vi "saveTetTaskToMAX..vi"() -> ()   [LabVIEW 2010]
doc: "Author: Mani Subramaniyan\n2011-09-14\n\nThis vi assumes you have 7, 4498 cards for recording from tetrodes."
uses:
  <vilib>/DAQmx/create/channels.llb/DAQmx Create Channel (AI-Voltage-Basic).vi
  <vilib>/DAQmx/configure/timing.llb/DAQmx Timing (Sample Clock).vi
  <vilib>/imath/engines/lvmath2/RunTimeEngine/ErrorHandling/NIMS_Finalize Error.vi
  <vilib>/imath/engines/lvmath2/RunTimeEngine/RangeToken/NIMS_Range_R2 - Integer.vi
  <instcachedir>/0/NIMS_Range_R2 - Integer_217CA55F27D14E80B3D190635C7B3F47.lvgen/NIMS_Range_R2 - Integer_217CA55F27D14E80B3D190635C7B3F47_000.vi
  <vilib>/imath/engines/lvmath2/RunTimeEngine/NodeEndStatement/NIMS_NodeEndStatement_Output.vi
  <instcachedir>/0/NIMS_NodeEndStatement_Output_53EC0D466D134D7ABD903AC30B43404B.lvgen/NIMS_NodeEndStatement_Output_53EC0D466D134D7ABD903AC30B43404B_004.vi
  <vilib>/imath/engines/lvmath2/RunTimeEngine/CommandStatement/MC_CommandStatement_break.vi
  <vilib>/imath/engines/lvmath2/RunTimeEngine/VariableToken/NIMS_VariableToken_CondDefinedDefinedByReplace.vi
  <instcachedir>/0/NIMS_VariableToken_CondDefinedDefinedByReplace_D162CFFC24174562A9FEA619A91E1A56.lvgen/NIMS_VariableToken_CondDefinedDefinedByReplace_D162CFFC24174562A9FEA619A91E1A56_003.vi
  <vilib>/imath/engines/lvmath2/RunTimeEngine/ReplaceToken/NIMS_Replace - Check Linear.vi
  <instcachedir>/0/NIMS_Replace - Check Linear_662D5651E4E34E0584DA82A256193A4C.lvgen/NIMS_Replace - Check Linear_662D5651E4E34E0584DA82A256193A4C_006.vi
  <vilib>/imath/engines/lvmath2/RunTimeEngine/ReplaceToken/NIMS_Replace - Size Check _(_)=S.vi
  <instcachedir>/0/NIMS_Replace - Size Check _(_)=S_6CAC13ACC74349C582FDAB09BCDAB70F.lvgen/NIMS_Replace - Size Check _(_)=S_6CAC13ACC74349C582FDAB09BCDAB70F_005.vi
  <vilib>/imath/engines/lvmath2/RunTimeEngine/ReplaceToken/NIMS_Replace - V(S)=S.vi
  <instcachedir>/0/NIMS_Replace - V(S)=S_78FDB6CCD265407D8926E4CF958018EB.lvgen/NIMS_Replace - V(S)=S_78FDB6CCD265407D8926E4CF958018EB_003.vi
  <vilib>/imathl/engines/lvmath/Functions/Error Handling/Create Error.vi
  <instcachedir>/0/NIMS_VariableToken_CondDefinedDefinedByReplace_D162CFFC24174562A9FEA619A91E1A56.lvgen/NIMS_VariableToken_CondDefinedDefinedByReplace_D162CFFC24174562A9FEA619A91E1A56_002.vi
  <instcachedir>/0/NIMS_Replace - Check Linear_662D5651E4E34E0584DA82A256193A4C.lvgen/NIMS_Replace - Check Linear_662D5651E4E34E0584DA82A256193A4C_005.vi
  <vilib>/imath/engines/lvmath2/RunTimeEngine/VariableToken/Read/NIMS_Get Elements - SorM(_,_) - Check - Check.vi
  <instcachedir>/0/NIMS_Get Elements - SorM(_,_) - Check - Check_507509EC3FB3473FB85D8EE7246D3CED.lvgen/NIMS_Get Elements - SorM(_,_) - Check - Check_507509EC3FB3473FB85D8EE7246D3CED_005.vi
  <instcachedir>/0/NIMS_Replace - Size Check _(_)=S_6CAC13ACC74349C582FDAB09BCDAB70F.lvgen/NIMS_Replace - Size Check _(_)=S_6CAC13ACC74349C582FDAB09BCDAB70F_004.vi
  <instcachedir>/0/NIMS_Replace - V(S)=S_78FDB6CCD265407D8926E4CF958018EB.lvgen/NIMS_Replace - V(S)=S_78FDB6CCD265407D8926E4CF958018EB_002.vi
  <vilib>/imath/engines/lvmath2/RunTimeEngine/ErrorHandling/NIMS_Create Error From Enums.vi
  <vilib>/imath/engines/lvmath2/RunTimeEngine/VariableToken/NIMS_VariableToken_CondDefined.vi
  <instcachedir>/0/NIMS_VariableToken_CondDefined_40F5A17402C24691AFAF09F6009BF744.lvgen/NIMS_VariableToken_CondDefined_40F5A17402C24691AFAF09F6009BF744_004.vi
  <instcachedir>/0/NIMS_VariableToken_CondDefined_40F5A17402C24691AFAF09F6009BF744.lvgen/NIMS_VariableToken_CondDefined_40F5A17402C24691AFAF09F6009BF744_003.vi
  <vilib>/imath/engines/lvmath2/RunTimeEngine/BuiltInFunctions/transpose/NIMS_transpose(GM).vi
  <instcachedir>/0/NIMS_transpose(GM)_822C4B39CC3F4B34B360A85316D387F1.lvgen/NIMS_transpose(GM)_822C4B39CC3F4B34B360A85316D387F1_003.vi
  <vilib>/imath/engines/lvmath2/RunTimeEngine/VariableToken/Read/NIMS_Get Elements - M($).vi
  <instcachedir>/0/NIMS_Get Elements - M($)_A8F2A19C5154485F939AC006E49BBA6A.lvgen/NIMS_Get Elements - M($)_A8F2A19C5154485F939AC006E49BBA6A_004.vi
  <vilib>/imath/engines/lvmath2/RunTimeEngine/VariableToken/Read/NIMS_Get Elements - CV(_) - Check(_).vi
  <instcachedir>/0/NIMS_Get Elements - CV(_) - Check(_)_64AEF14B7A4641C2943F7B5E6C404257.lvgen/NIMS_Get Elements - CV(_) - Check(_)_64AEF14B7A4641C2943F7B5E6C404257_001.vi
  <instcachedir>/0/NIMS_Get Elements - CV(_) - Check(_)_64AEF14B7A4641C2943F7B5E6C404257.lvgen/NIMS_Get Elements - CV(_) - Check(_)_64AEF14B7A4641C2943F7B5E6C404257_000.vi
  <vilib>/imath/engines/lvmath2/RunTimeEngine/BuiltInFunctions/sort/NIMS_[2o]_sort(RColV,I32,Str).vi
  <instcachedir>/0/NIMS_[2o]_sort(RColV,I32,Str)_8C46B823F3A24849A9EF3A3AB0F8B237.lvgen/NIMS_[2o]_sort(RColV,I32,Str)_8C46B823F3A24849A9EF3A3AB0F8B237_001.vi
  <vilib>/imath/engines/lvmath2/RunTimeEngine/VariableToken/Read/NIMS_Get Elements - CV(_) - Check.vi
  <instcachedir>/0/NIMS_Get Elements - CV(_) - Check_8515505E2F3A4209803E127475018AE3.lvgen/NIMS_Get Elements - CV(_) - Check_8515505E2F3A4209803E127475018AE3_001.vi
  <vilib>/imath/engines/lvmath2/RunTimeEngine/BuiltInFunctions/ones/NIMS_V=ones(I32,I32).vi
  <vilib>/imath/engines/lvmath2/RunTimeEngine/RangeToken/NIMS_Range.vi
  <instcachedir>/0/NIMS_Range_1C63927E4E474DADACDA97C3F2261A11.lvgen/NIMS_Range_1C63927E4E474DADACDA97C3F2261A11_000.vi
  <vilib>/imath/engines/lvmath2/RunTimeEngine/BuiltInFunctions/repeatmx/NIMS_repeatmx(GM, I32, I32).vi
  <instcachedir>/0/NIMS_repeatmx(GM, I32, I32)_69DEE8FEFC4F4D9AB51BA55E85245ECE.lvgen/NIMS_repeatmx(GM, I32, I32)_69DEE8FEFC4F4D9AB51BA55E85245ECE_004.vi
  <instcachedir>/0/NIMS_Get Elements - M($)_A8F2A19C5154485F939AC006E49BBA6A.lvgen/NIMS_Get Elements - M($)_A8F2A19C5154485F939AC006E49BBA6A_005.vi
  <instcachedir>/0/NIMS_Get Elements - CV(_) - Check_8515505E2F3A4209803E127475018AE3.lvgen/NIMS_Get Elements - CV(_) - Check_8515505E2F3A4209803E127475018AE3_003.vi
panel:
  in  "Stop Without Saving":bool
  in  "Deselect All":bool
  in  "Save Task Now":bool
  in  "Select All":bool
  out "error out":errorcluster
  in  "Sampling Rate (Hz)":dbl=32000.0 format="%0.2f"
  out "Channel Names":string[](array[string])=["t10c4", "t1c4", "t10c3", "t1c3", "t10c2", "t1c2", "t10c1", "t1c1", "t11c4", "t2c4", "t11c3", "t2c3", "t11c2", "t2c2", "t11c1", "t2c1", "t3c4", "t12c4", "t3c3", "t12c3", "t3c2", "t12c2", "t3c1", "t12c1", "t4c4", "t7c4", "t4c3", "t7c3", "t4c2", "t7c2", "t4c1", "t7c1", "t5c4", "t8c4", "t5c3", "t8c3", "t5c2", "t8c2", "t5c1", "t8c1", "t9c4", "t6c4", "t9c3", "t6c3", "t9c2", "t6c2", "t9c1", "t6c1", "t13c4", "t13c3", "t13c2", "t13c1", "t14c4", "t14c3", "t14c2", "t14c1", "t15c4", "t15c3", "t15c2", "t15c1"]
  out "Physical Channels":string[](array[string])=["4498_1/ai0", "4498_1/ai1", "4498_1/ai2", "4498_1/ai3", "4498_1/ai4", "4498_1/ai5", "4498_1/ai6", "4498_1/ai7", "4498_1/ai8", "4498_1/ai9", "4498_1/ai10", "4498_1/ai11", "4498_1/ai12", "4498_1/ai13", "4498_1/ai14", "4498_1/ai15", "4498_2/ai0", "4498_2/ai1", "4498_2/ai2", "4498_2/ai3", "4498_2/ai4", "4498_2/ai5", "4498_2/ai6", "4498_2/ai7", "4498_2/ai8", "4498_2/ai9", "4498_2/ai10", "4498_2/ai11", "4498_2/ai12", "4498_2/ai13", "4498_2/ai14", "4498_2/ai15", "4498_3/ai0", "4498_3/ai1", "4498_3/ai2", "4498_3/ai3", "4498_3/ai4", "4498_3/ai5", "4498_3/ai6", "4498_3/ai7", "4498_3/ai8", "4498_3/ai9", "4498_3/ai10", "4498_3/ai11", "4498_3/ai12", "4498_3/ai13", "4498_3/ai14", "4498_3/ai15", "4498_4/ai1", "4498_4/ai3", "4498_4/ai5", "4498_4/ai7", "4498_4/ai9", "4498_4/ai11", "4498_4/ai13", "4498_4/ai15", "4498_5/ai0", "4498_5/ai2", "4498_5/ai4", "4498_5/ai6"]
  in  "Task Name":string="untitled"
  in  "minimum value":dbl=-0.3
  in  "maximum value":dbl=0.3
  in  "1-4 Channels":bool[][](array[boolean])
  in  "Channel Mapping":u32[][](array[numeric])=[[7, 5, 3, 1], [15, 13, 11, 9], [22, 20, 18, 16], [30, 28, 26, 24], [38, 36, 34, 32], [47, 45, 43, 41], [31, 29, 27, 25], [39, 37, 35, 33], [46, 44, 42, 40], [6, 4, 2, 0], [14, 12, 10, 8], [23, 21, 19, 17], [55, 53, 51, 49], [63, 61, 59, 57], [70, 68, 66, 64], [78, 76, 74, 72], [86, 84, 82, 80], [95, 93, 91, 89], [79, 77, 75, 73], [87, 85, 83, 81], [94, 92, 90, 88], [54, 52, 50, 48], [62, 60, 58, 56], [71, 69, 67, 65], [96, 97, 98, 99], [103, 102, 101, 100], [104, 105, 106, 107], [108, 109, 110, 111]]
  # "Select Tetrode Channels For Task"
  # "1"
  # "1\n2\n3\n4\n5\n6\n7\n8\n9\n10\n11\n12\n13\n14\n15\n16\n17\n18\n19\n20\n21\n22\n23\n24\n25\n26\n27\n28"
  # "2"
  # "3"
  # "4"
  # "5"
  # "6"
  # "7"
  # "8"
  # "9"
  # "10"
  # "11"
  # "12"
  # "13"
  # "14"
  # "15"
  # "16"
  # "17"
  # "18"
  # "19"
  # "20"
  # "21"
  # "22"
  # "23"
  # "24"
  # "25"
  # "26"
  # "27"
  # "28"
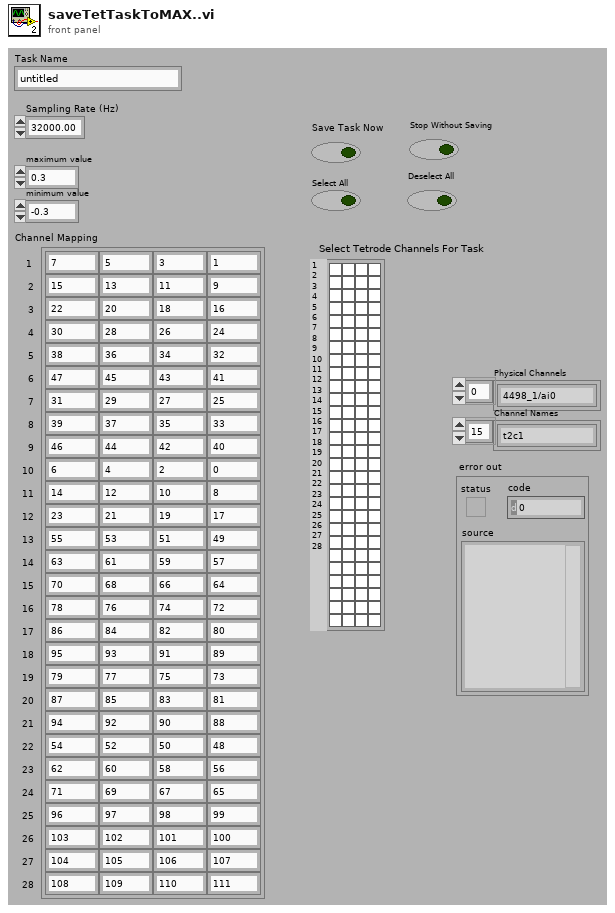
[diagram p1: front panel]
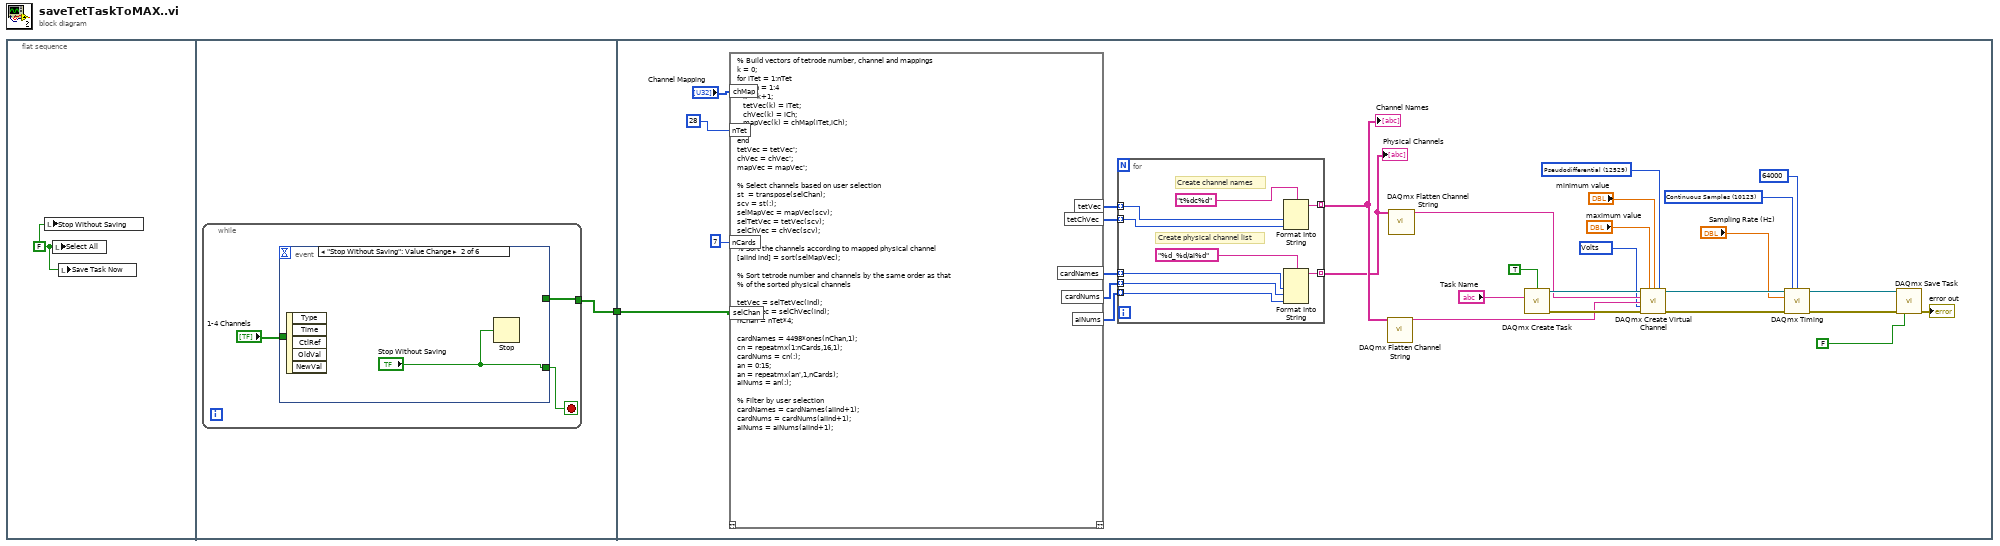
[diagram p0: block diagram]
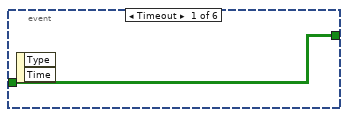
[diagram p2: hidden frame]
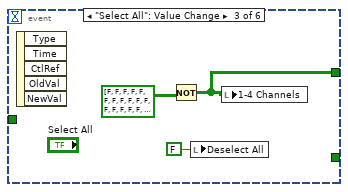
[diagram p3: hidden frame]
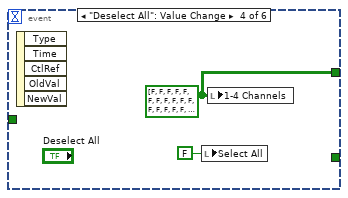
[diagram p4: hidden frame]
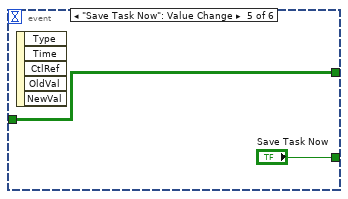
[diagram p5: hidden frame]
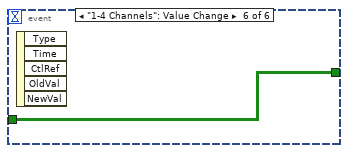
[diagram p6: hidden frame]
diagram:
  n1 = flat-sequence {
    tunnel: [w3] -> w1
    tunnel: w1 -> [w18]
    frame #0 {
      w2 = FALSE ("Select All")
      n2 = local write "Stop Without Saving"(w2) -> ()
      n3 = local write "Select All"(w2) -> ()
      n4 = local write "Save Task Now"(w2) -> ()
    }
    frame #1 {
      n5 = while {
        tunnel: [w5] -> w3
        stop <- w4 stop-if-true
        n6 = event shown="[1] \"Stop Without Saving\": Value Change" {
          selector: _ -> [_ _ _ _ _ _]
          dyn-events: _ -> [_ _ _ _ _ _]
          timeout: _ -> [_ _ _ _ _ _]
          tunnel: "1-4 Channels" -> [w7 _ _ _ w14 w16]
          tunnel: [w7 _ w9 w12 w14 w16] -> w5
          tunnel: [_ "Stop Without Saving" _ _ "Save Task Now" _] -> w4
          event Timeout {
            n7 = event-data() -> ()  [unwired: 1 in, 2 out]
          }
          event "Stop Without Saving": Value Change {
            n8 = event-data() -> ()  [unwired: 1 in, 5 out]
            n9 = Stop(stop? (T)="Stop Without Saving") -> ()
          }
          event "Select All": Value Change {
            n10 = event-data() -> ()  [unwired: 1 in, 5 out]
            n11 = Not(x=bool[][] [[FALSE, FALSE, FALSE, FALSE], [FALSE, FALSE, FALSE, FALSE], [FALSE, FALSE, FALSE, FALSE], [FALSE, FALSE, FALSE, FALSE], [FALSE, FALSE, FALSE, FALSE], [FALSE, FALSE, FALSE, FALSE], [FALSE, FALSE, FALSE, FALSE], [FALSE, FALSE, FALSE, FALSE], [FALSE, FALSE, FALSE, FALSE], [FALSE, FALSE, FALSE, FALSE], [FALSE, FALSE, FALSE, FALSE], [FALSE, FALSE, FALSE, FALSE], [FALSE, FALSE, FALSE, FALSE], [FALSE, FALSE, FALSE, FALSE], [FALSE, FALSE, FALSE, FALSE], [FALSE, FALSE, FALSE, FALSE], [FALSE, FALSE, FALSE, FALSE], [FALSE, FALSE, FALSE, FALSE], [FALSE, FALSE, FALSE, FALSE], [FALSE, FALSE, FALSE, FALSE], [FALSE, FALSE, FALSE, FALSE], [FALSE, FALSE, FALSE, FALSE], [FALSE, FALSE, FALSE, FALSE], [FALSE, FALSE, FALSE, FALSE], [FALSE, FALSE, FALSE, FALSE], [FALSE, FALSE, FALSE, FALSE], [FALSE, FALSE, FALSE, FALSE], [FALSE, FALSE, FALSE, FALSE]] ("1-4 Channels")) -> (.not. x?=w9:bool[][])
            n12 = local write "Deselect All"(FALSE ("Deselect All")) -> ()
            n13 = local write "1-4 Channels"(w9) -> ()
          }
          event "Deselect All": Value Change {
            w12 = bool[][] [[FALSE, FALSE, FALSE, FALSE], [FALSE, FALSE, FALSE, FALSE], [FALSE, FALSE, FALSE, FALSE], [FALSE, FALSE, FALSE, FALSE], [FALSE, FALSE, FALSE, FALSE], [FALSE, FALSE, FALSE, FALSE], [FALSE, FALSE, FALSE, FALSE], [FALSE, FALSE, FALSE, FALSE], [FALSE, FALSE, FALSE, FALSE], [FALSE, FALSE, FALSE, FALSE], [FALSE, FALSE, FALSE, FALSE], [FALSE, FALSE, FALSE, FALSE], [FALSE, FALSE, FALSE, FALSE], [FALSE, FALSE, FALSE, FALSE], [FALSE, FALSE, FALSE, FALSE], [FALSE, FALSE, FALSE, FALSE], [FALSE, FALSE, FALSE, FALSE], [FALSE, FALSE, FALSE, FALSE], [FALSE, FALSE, FALSE, FALSE], [FALSE, FALSE, FALSE, FALSE], [FALSE, FALSE, FALSE, FALSE], [FALSE, FALSE, FALSE, FALSE], [FALSE, FALSE, FALSE, FALSE], [FALSE, FALSE, FALSE, FALSE], [FALSE, FALSE, FALSE, FALSE], [FALSE, FALSE, FALSE, FALSE], [FALSE, FALSE, FALSE, FALSE], [FALSE, FALSE, FALSE, FALSE]] ("1-4 Channels")
            n14 = event-data() -> ()  [unwired: 1 in, 5 out]
            n15 = local write "Select All"(FALSE ("Select All")) -> ()
            n16 = local write "1-4 Channels"(w12) -> ()
          }
          event "Save Task Now": Value Change {
            n17 = event-data() -> ()  [unwired: 1 in, 5 out]
          }
          event "1-4 Channels": Value Change {
            n18 = event-data() -> ()  [unwired: 1 in, 5 out]
          }
        }
      }
    }
    frame #2 {
      w20 = 12529 items=["default"=-1, "RSE"=10083, "NRSE"=10078, "Differential"=10106, "Pseudodifferential"=12529] ("input terminal configuration")
      w26 = 10123 items=["Finite Samples"=10178, "Continuous Samples"=10123, "Hardware Timed Single Point"=12522] ("sample mode")
      w29 = 10348 items=["Volts"=10348, "From Custom Scale"=10065] ("units")
      n19 = mathscript code="% Build vectors of tetrode number, channel and mappings\nk = 0;\nfor iTet = 1:nTet\nfor iCh = 1:4\n   k = k+1;\n   tetVec(k) = iTet;\n   chVec(k) = iCh;\n   mapVec(k) = chMap(iTet,iCh);\nend\nend\ntetVec = tetVec';\nchVec = chVec';\nmapVec = mapVec';\n\n% Select channels based on user selection\nst  = transpose(selChan);\nscv = st(:);\nselMapVec = mapVec(scv);\nselTetVec = tetVec(scv);\nselChVec = chVec(scv);\n\n% Sort the channels according to mapped physical channel\n[aiInd ind] = sort(selMapVec);\n\n% Sort tetrode number and channels by the same order as that\n% of the sorted physical channels\n\ntetVec = selTetVec(ind);\ntetChVec = selChVec(ind);\nnChan = nTet*4;\n\ncardNames = 4498*ones(nChan,1);\ncn = repeatmx(1:nCards,16,1);\ncardNums = cn(:);\nan = 0:15;\nan = repeatmx(an',1,nCards);\naiNums = an(:);\n\n% Filter by user selection\ncardNames = cardNames(aiInd+1);\ncardNums = cardNums(aiInd+1);\naiNums = aiNums(aiInd+1);"("chMap"="Channel Mapping", "nTet"=u32 28 ("dimension size"), "nCards"=u32 7 ("dimension size"), "selChan"=w18) -> ("tetVec"=w40:i32[], "tetChVec"=w39:i32[], "cardNames"=w43:i32[], "cardNums"=w42:i32[], "aiNums"=w41:i32[])  [unwired: 1 in, 1 out]
      n20 = for {
        tunnel: w43 -> [w55] mode=indexing
        tunnel: w42 -> [w54] mode=indexing
        tunnel: w41 -> [w53] mode=indexing
        tunnel: [w51] -> w31 mode=indexing
        tunnel: w40 -> [w50] mode=indexing
        tunnel: w39 -> [w49] mode=indexing
        tunnel: [w47] -> w33 mode=indexing
        # "Create channel names"
        # "Create physical channel list"
        n21 = Format Into String(format string="t%dc%d", w50, w49) -> (resulting string=w47:string)  [unwired: 2 in, 1 out]
        n22 = Format Into String(format string="%d_%d/ai%d", w55, w54, w53) -> (resulting string=w51:string)  [unwired: 2 in, 1 out]
      }
      "Physical Channels" <- w31
      "Channel Names" <- w33
      n23 = call <vilib>:"DAQmx Flatten Channel String.vi"("names in"=w33) -> ("names out"=w32:string)  [unwired: 13 in, 1 out]
      n24 = call <vilib>:"DAQmx Flatten Channel String.vi"("names in"=w31) -> ("names out"=w30:string)  [unwired: 13 in, 1 out]
      n25 = call <vilib>:"DAQmx Create Task.vi"("new task name"="Task Name", "auto cleanup"=TRUE) -> ("task out"=w34:refnum<k21>, "error out"=w35:errorcluster)  [unwired: 12 in]
      n26 = call-poly <vilib>:"DAQmx Create Virtual Channel.vi"("task in"=w34, "maximum value"="maximum value", "minimum value"="minimum value", "input terminal configuration"=w20, "physical channels"=w30, "name to assign"=w32, "units"=w29, "error in"=w35) -> ("task out"=w28:refnum<k21>, "error out"=w22:errorcluster)  [unwired: 6 in]
      n27 = call-poly <vilib>:"DAQmx Timing.vi"("task/channels in"=w28, "sample mode"=w26, "samples per channel"=64000, "rate"="Sampling Rate (Hz)", "error in"=w22) -> ("task out"=w24:refnum<k21>, "error out"=w21:errorcluster)  [unwired: 9 in]
      n28 = call <vilib>:"DAQmx Save Task.vi"("task/channels in"=w24, "error in"=w21, "overwrite existing task?"=FALSE) -> ("error out"=→"error out":errorcluster)  [unwired: 11 in, 1 out]
    }
  }
